vi "KVP to Variant.vi"(9 "Cluster Name":string="untitled") -> (2 "Reconstructed Data":variant, 10 "KVP":variant)   [LabVIEW 2013]
doc: "This VI takes a default value as the input and replaces it recursively (cluster, array) with values found in key value pair arrays."
uses:
  <vilib>/Utility/GetType.llb/TD_Create Cluster.vi
  Variant/OpenVariant.lvlib
panel:
  out "names":string[](array[string])
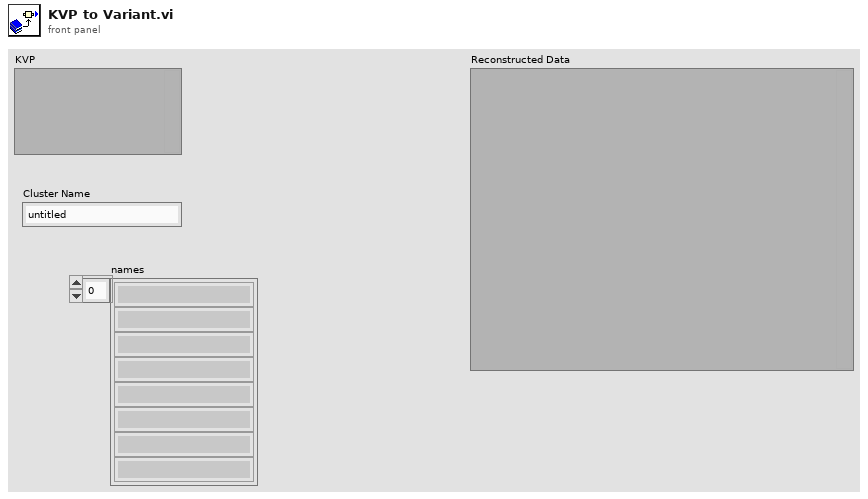
[diagram p1: front panel]
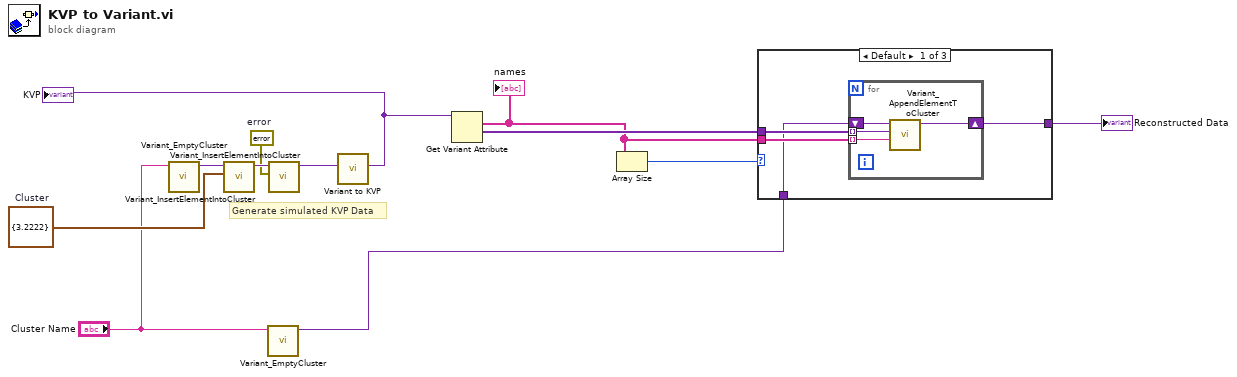
[diagram p0: block diagram]
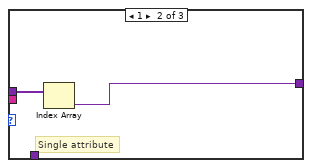
[diagram p2: hidden frame]
diagram:
  w7 = cluster{"test":dbl} {"test"=3.2222}  # Cluster
  w5 = errorcluster {"status"=FALSE, "code"=42, "source"="fgjksfrjsfgk"}  # error
  # "Generate simulated KVP Data"
  n1 = call "Variant_EmptyCluster.vi"("Cluster Name"="Cluster Name") -> ("Empty Cluster"=w8:variant)  [unwired: 10 in]
  n2 = call "Variant_InsertElementIntoCluster.vi"("Element"=w7, "Cluster in"=w8) -> ("Cluster out"=w6:variant)  [unwired: 9 in]
  n3 = call "Variant_EmptyCluster.vi"("Cluster Name"="Cluster Name") -> ("Empty Cluster"=w9:variant)  [unwired: 10 in]
  n4 = call "Variant_InsertElementIntoCluster.vi"("Element"=w5, "Cluster in"=w6) -> ("Cluster out"=w4:variant)  [unwired: 9 in]
  n5 = call "Variant to KVP.vi"("Variant"=w4) -> ("KVP"=w2:variant)  [unwired: 10 in]
  "KVP" <- w2
  n6 = Get Variant Attribute(Variant=w2) -> (names=w10:string[], values=w12:variant[])  [unwired: 3 in, 2 out]
  "names" <- w10
  n7 = Array Size(array=w10) -> (size(s)=w11:i32)
  n8 = case shown="Default" w11 {
    tunnel: w12 -> [w15 w22 _]
    tunnel: w10 -> [w16 _ _]
    tunnel: [w14 w21 _] -> w3
    tunnel: w9 -> [w13 _ _]
    frame Default {
      n9 = for {
        tunnel: w16 -> [w17] mode=indexing
        tunnel: w15 -> [w20] mode=indexing
        shift-right: [w18] -> w14
        shift-left: w13 -> [w19]
        n10 = call "Variant_AppendElementToCluster.vi"("Element name"=w17, "Element"=w20, "Data in"=w19) -> ("Data out"=w18:variant)  [unwired: 8 in]
      }
    }
    frame 1 {
      # "Single attribute"
      n11 = Index Array(array=w22) -> (element=w21:variant)  [unwired: 1 in]
    }
    frame 0 {
    }
  }
  "Reconstructed Data" <- w3
